vi "Check Temp Stable.vi"(8 "timeperiod":dbl=20.0, 9 "sens":dbl=0.05, 11 "temparray":dbl[](array[numeric])) -> (0 "stable":bool)   [LabVIEW 2015, in "Temperature Controller.lvclass"]
uses:
  Temperature Controller.lvclass
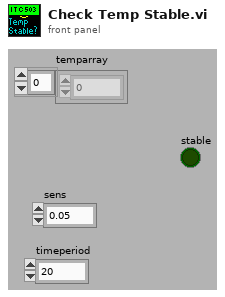
[diagram p1: front panel]
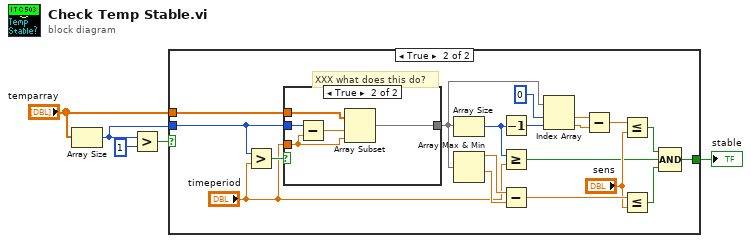
[diagram p0: block diagram]
diagram:
  n1 = Array Size(array="temparray") -> (size(s)=w3:i32)
  n2 = Greater?(x=w3, y=1) -> (0:w4:bool)
  n3 = case shown="True" w4 {
    tunnel: "temparray" -> [_ w20]
    tunnel: w3 -> [_ w19]
    tunnel: [_ w13] -> w5
    frame False {
    }
    frame True {
      # "XXX what does this do?"
      n4 = Greater?(x=w19, y="timeperiod") -> (0:w21:bool)
      n5 = case shown="True" w21 {
        tunnel: w20 -> [w25 w30]
        tunnel: "timeperiod" -> [_ w27]
        tunnel: w19 -> [_ w29]
        tunnel: [w25 w26] -> w17
        frame False {
        }
        frame True {
          n6 = Subtract(x=w29, y=w27) -> (x-y=w28:dbl)
          n7 = Array Subset(array=w30, index=w28, length=w27) -> (w26:dbl[])
        }
      }
      n8 = Array Size(array=w17) -> (size(s)=w15:i32)
      n9 = Array Max & Min(array=w17) -> (max value=w24:dbl, min value=w23:dbl)  [unwired: 2 out]
      n10 = Decrement(x=w15) -> (x-1=w14:i32)
      n11 = Greater Or Equal?(x=w15, y="timeperiod") -> (x >= y?=w7:bool)
      n12 = Subtract(x=w24, y=w23) -> (x-y=w22:dbl)
      n13 = Index Array(array=w17, index #1=0, index #2=w14) -> (element #1=w12:dbl, element #2=w11:dbl)
      n14 = Subtract(x=w12, y=w11) -> (x-y=w10:dbl)
      n15 = Less Or Equal?(x=w10, y="sens") -> (x <= y?=w8:bool)
      n16 = Less Or Equal?(x=w22, y="sens") -> (x <= y?=w6:bool)
      n17 = Compound Arithmetic op=AND(w8, w7, w6) -> (w13:bool)
    }
  }
  "stable" <- w5
